vi "GSP_Manager_GT.vi"() -> ()   [LabVIEW 2015]
uses:
  SystemUtil/Command.ctl
  SystemUtil/ScriptArray.ctl
  SystemUtil/Script.ctl
  SystemUtil/MotorStates.ctl
  SystemUtil/ThreadStates.ctl
  Log/LogItem.ctl
  GSP_GT_Global.vi
  GUI/GSP_GUI_global.vi
panel:
  out "Gratings":T1(array[cluster])
  out "lines/mm":i32
  in  "Grating #":i32(ring) items=["<NO GRATING>", "SYZY_400", "RALC_1200", "SYZY_2100"]
  out "Last Error":errorcluster
  in  "CommandQ":string
  # "Grating"
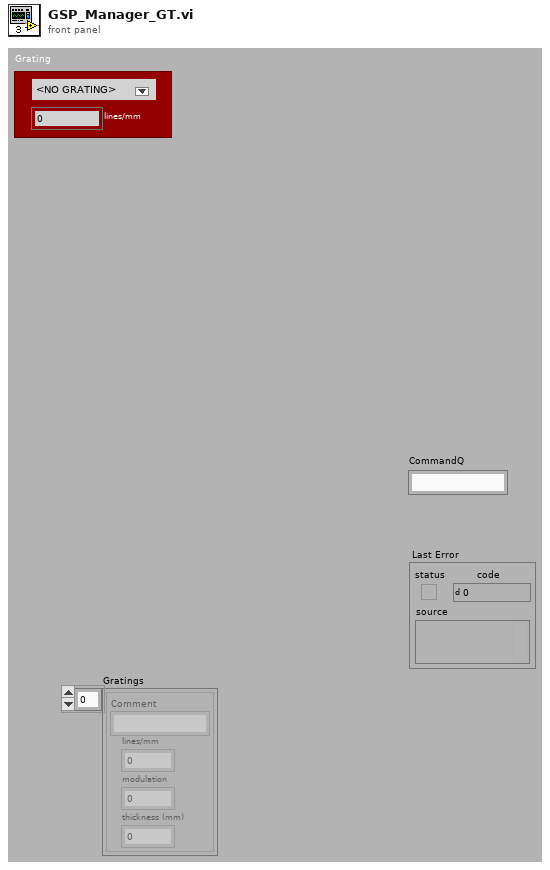
[diagram p1: front panel]
types:
  T1 = cluster{"Comment":string, "lines/mm":i32, "modulation":dbl, "thickness (mm)":dbl}[]
  T2 = typedef "Command.ctl" = cluster{"Command":string, "Parameter":string}
  T3 = typedef "ScriptArray.ctl" = T4[]
  T4 = typedef "Script.ctl" = cluster{"Current Step":i32, "Commands":cluster{"Command":string, "Parameters":string}[]}
  T5 = cluster{"Move Mem Address":i32, "Home Mem Address":i32}
  T6 = typedef "MotorStates.ctl" = enum16{"Ready", "Moving", "Uninitialized", "Error"}
  T7 = typedef "ThreadStates.ctl" = enum16{"Waiting", "Scripting", "Uninitialized", "Error"}
  T8 = cluster{"Comment":string, "lines/mm":i32, "modulation":dbl, "thickness (mm)":dbl}
  T9 = enum16{"Launch", "Log", "Open", "Close", "Shutdown"}
  T10 = typedef "LogItem.ctl" = cluster{"error in (no error)":errorcluster, "Source":string, "Comment ":string}
  T11 = enum16{"POL (0)", "CPL (1)", "HLT (2)", "STP (3)", "RST (4)", "RVN (5)", "RPB (6)", "CLP (8)", "SDL (9)", "RUN (10)", "WRI (11)", "RRG (12)", "SPR (13)", "LPR (14)", "VMI (15)", "SSP (17)", "SSE (18)", "RIS (20)", "RIO (21)", "IMW (25)", "END (128)", "MAV (134)", "MRV (135)", "JRE (137)", "WCL (138)", "WCW (139)", "DLY (140)", "WDL (141)", "GCL (142)", "GOP (143)", "ZTG (144)", "ZTP (145)", "TTP (146)", "CME (147)", "CTC (148)", "TQL (149)", "AHC (150)", "ERL (151)", "OLP (152)", "WRP (154)", "IDT (155)", "LRP (156)", "VMP (159)", "RAV (160)", "RRV (161)", "JMP (162)", "JOI (162)", "CIS (163)", "CKS (164)", "CLC (165)", "KMC (167)", "MCT (168)", "FLC (169)", "EEM (170)", "DDB (171)", "DEM (171)", "PAC (172)", "ADL (173)", "BRT (174)", "MAT (176)", "MRT (177)", "RAT (178)", "RRT (179)", "SSD (180)", "KMR (181)", "KED (182)", "KDD (183)", "DIR (184)", "PRO (185)", "SIF (186)", "EDL (187)", "CIO (188)", "MDS (189)", "MDC (190)", "MDT (191)", "SEE (192)", "ARI (193)", "WBS (194)", "SCF (195)", "RSM (196)", "RLM (197)", "RSN (198)", "RLN (199)", "PCL (201)", "PCI (201)", "PRT (202)", "PRI (202)", "WBE (204)", "SOB (205)", "COB (206)", "ACR (207)", "PLR (208)", "CAI (211)", "LVT (212)", "OVT (213)", "MTT (214)", "CLC (215)", "PIM (216)", "VIM (217)", "TIM (218)", "AHM (219)", "SSL (221)", "TRU (222)", "RSD (223)", "EMT (225)", "DMT (226)", "EMD (227)", "DMD (228)", "HSM (229)", "AHD (230)", "PCM (231)", "PCG (232)", "XRV (233)", "XAV (234)", "XRT (235)", "XAT (236)", "GOC (237)", "JNA (238)", "JOR (239)", "PMC (240)", "PMV (241)", "PMX (242)", "DLC (243)", "SLC (244)", "PCP (245)", "ATR (248)", "PMO (249)", "JAN (250)", "EDH (251)", "DIF (252)", "IMS (253)", "IMQ (254)"}
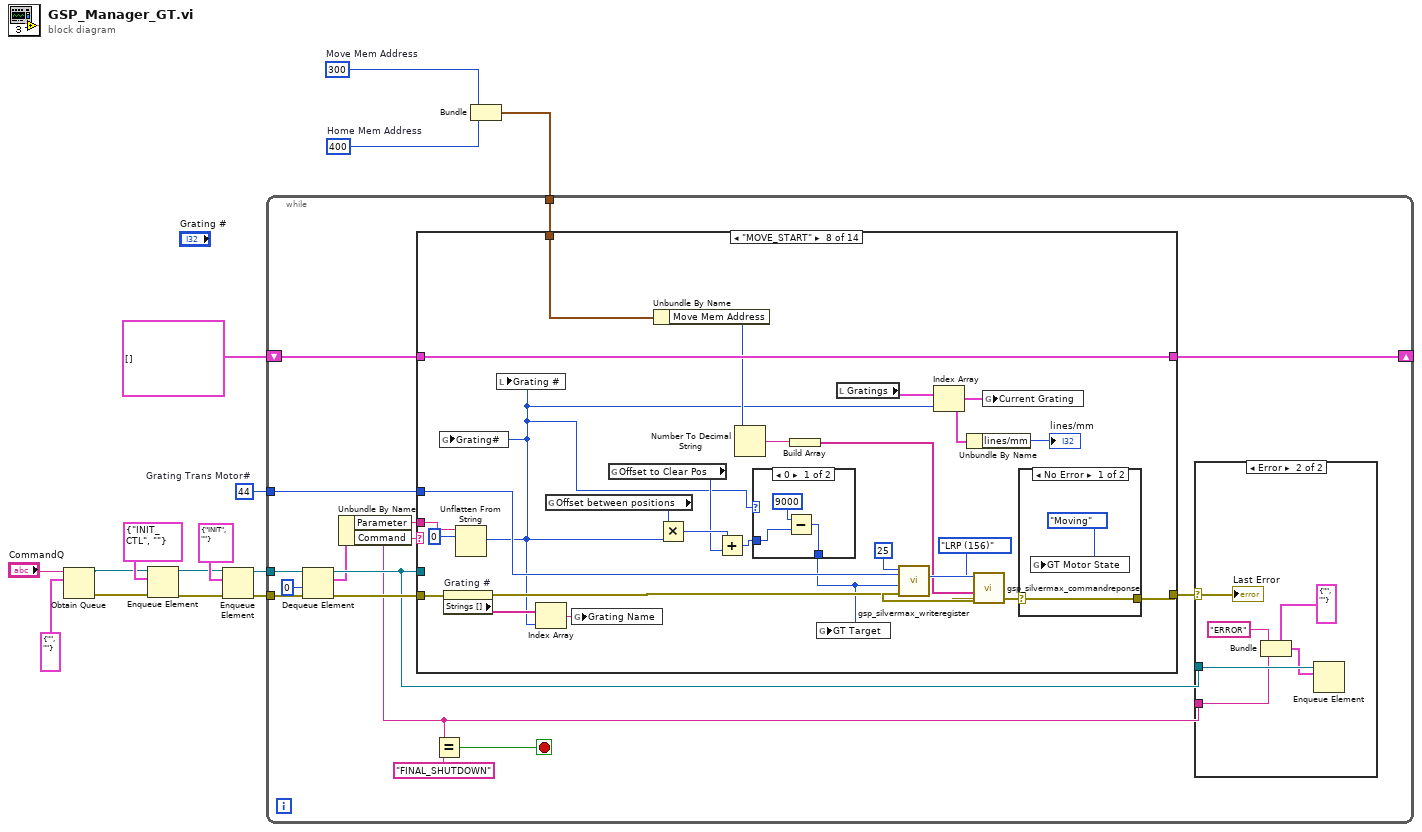
[diagram p0: block diagram]
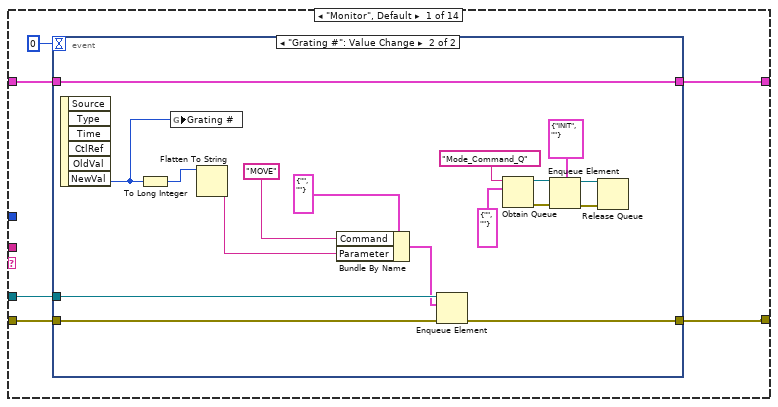
[diagram p3: hidden frame]
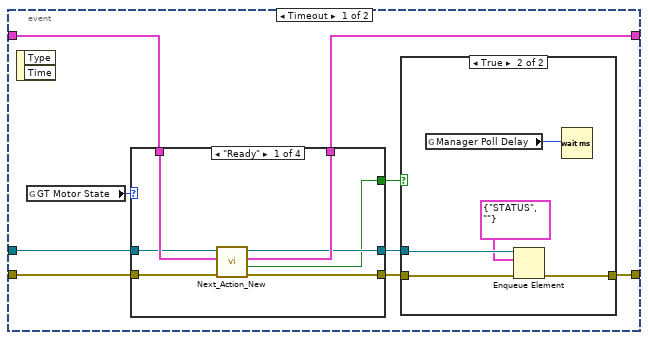
[diagram p4: hidden frame]
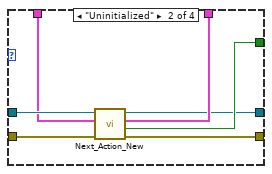
[diagram p6: hidden frame]
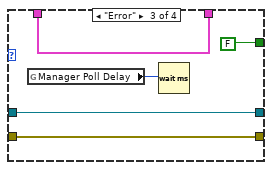
[diagram p7: hidden frame]
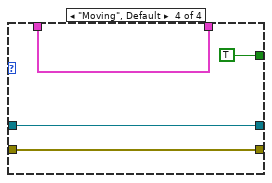
[diagram p8: hidden frame]
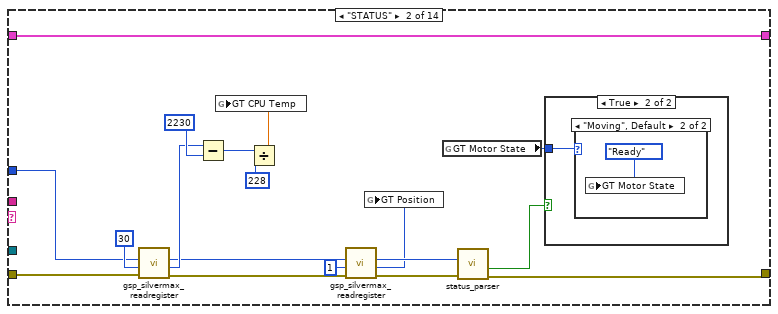
[diagram p9: hidden frame]
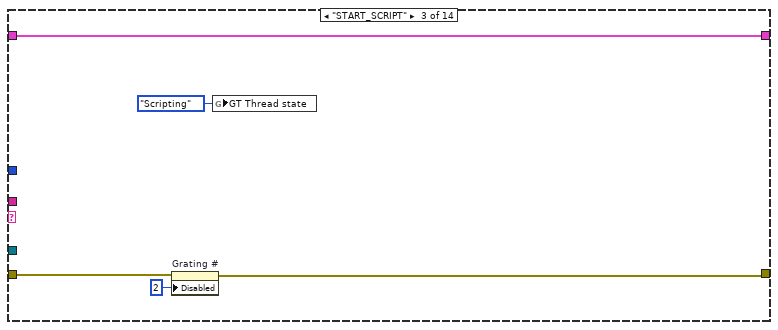
[diagram p12: hidden frame]
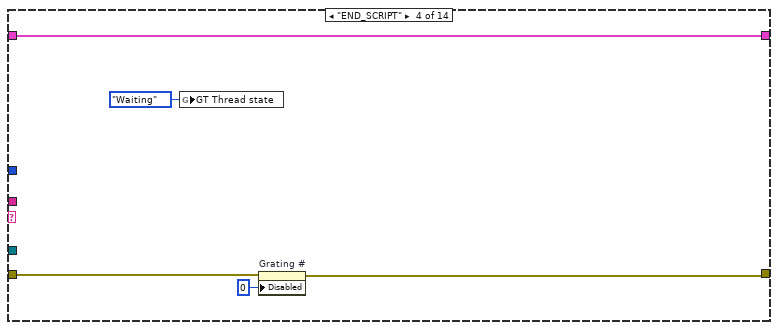
[diagram p13: hidden frame]
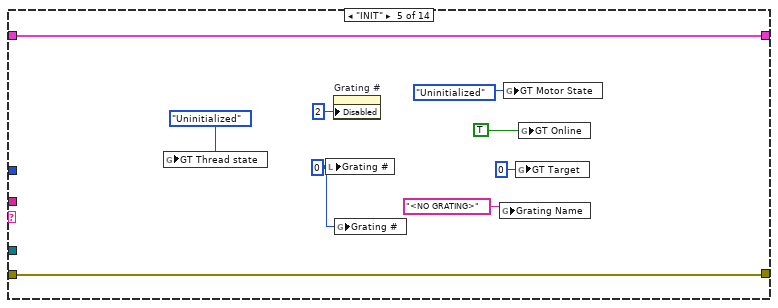
[diagram p14: hidden frame]
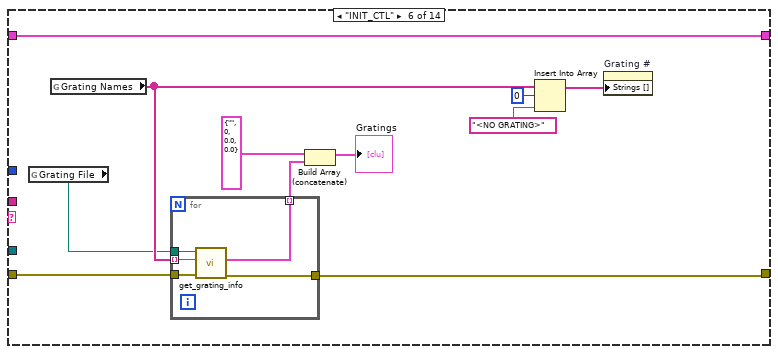
[diagram p15: hidden frame]
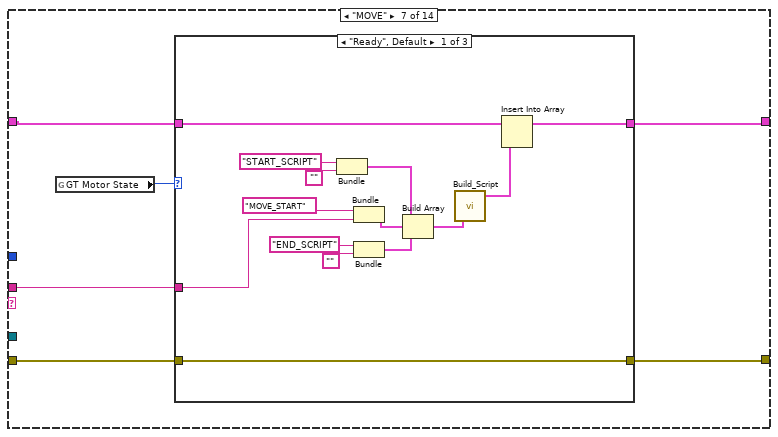
[diagram p16: hidden frame]
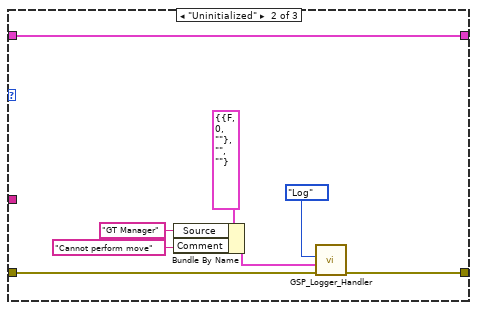
[diagram p17: hidden frame]
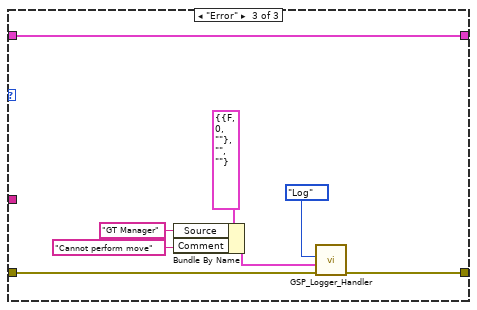
[diagram p18: hidden frame]
diagram:
  w7 = 400  # Home Mem Address
  w8 = 300  # Move Mem Address
  w9 = u8 44  # Grating Trans Motor#
  n1 = Obtain Queue(name (unnamed)="CommandQ", element data type=T2 {"Command"="", "Parameter"=""} ("Command")) -> (queue out=w2:refnum<queue>, error out=w1:errorcluster)  [unwired: 3 in, 1 out]
  n2 = Enqueue Element(queue=w2, element=T2 {"Command"="INIT_CTL", "Parameter"=""}, error in (no error)=w1) -> (queue out=w4:refnum<queue>, error out=w3:errorcluster)  [unwired: 1 in, 1 out]
  n3 = Enqueue Element(queue=w4, element=T2 {"Command"="INIT", "Parameter"=""}, error in (no error)=w3) -> (queue out=w15:refnum<queue>, error out=w14:errorcluster)  [unwired: 1 in, 1 out]
  n4 = Bundle("Move Mem Address"=w8, "Home Mem Address"=w7) -> (w6:T5)  [unwired: 1 in]
  n5 = while {
    tunnel: w15 -> [w30]
    tunnel: w14 -> [w29]
    tunnel: w9 -> [w24]
    shift-right: [w18] -> _
    shift-left: T3 [] ("Operations") -> [w23]
    tunnel: w6 -> [w16]
    stop <- w19 stop-if-true
    n6 = Dequeue Element(queue=w30, timeout in ms (-1)=0, error in (no error)=w29) -> (queue out=w26:refnum<queue>, element=w21:T2, error out=w28:errorcluster)  [unwired: 1 out]
    n7 = Unbundle By Name(w21) -> ("Parameter"=w17:string, "Command"=w20:string)
    n8 = case shown="\"MOVE_START\"" w20 {
      tunnel: w28 -> [w41 w106 w120 w126 w132 w140 w155 w195 w229 w248 w283 w302 w304 _]
      tunnel: w26 -> [w42 _ _ _ _ _ _ _ _ w251 w282 _ _ w326]
      tunnel: [w38 w115 w119 w125 w132 w143 w154 w209 w237 w250 w279 w302 w312 _] -> w27
      tunnel: w24 -> [_ w105 _ _ _ _ _ w212 w240 _ _ _ w314 _]
      tunnel: w23 -> [w40 w113 w122 w127 w135 w147 w158 w206 w234 w252 w281 w301 w309 w320]
      tunnel: [w39 w113 w122 w127 w135 w147 w157 w206 w234 w249 w281 w300 w309 w319] -> w18
      tunnel: w17 -> [_ _ _ _ _ _ w156 w205 _ _ _ _ _ _]
      tunnel: w16 -> [_ _ _ _ _ _ _ w200 w233 _ _ _ w307 _]
      frame "Monitor", Default {
        n9 = event shown="[1] \"Grating #\": Value Change" {
          selector: _ -> [_ _]
          dyn-events: _ -> [_ _]
          timeout: 0 -> [_ _]
          tunnel: w42 -> [w51 w90]
          tunnel: w41 -> [w50 w91]
          tunnel: w40 -> [w49 w97]
          tunnel: [w48 w97] -> w39
          tunnel: [w44 w92] -> w38
          event Timeout {
            n10 = event-data() -> ()  [unwired: 1 in, 2 out]
            n11 = global read "GSP_GT_Global.vi" "GT Motor State"() -> (w43:T6)
            n12 = case shown="\"Ready\"" w43 {
              tunnel: w51 -> [w60 w69 w73 w78]
              tunnel: w50 -> [w64 w71 w75 w79]
              tunnel: [w62 w70 w75 w79] -> w47
              tunnel: w49 -> [w61 w68 w74 w80]
              tunnel: [w63 w67 w74 w80] -> w48
              tunnel: [w59 w65 w73 w78] -> w46
              tunnel: [w58 w66 FALSE TRUE] -> w45
              frame "Ready" {
                n13 = call "Next_Action_New.vi"("error in (no error)"=w64, "Operations"=w61, "queue in"=w60) -> ("error out"=w62:errorcluster, "No command?"=w58:bool, "Operations Out"=w63:T3, "queue out"=w59:refnum<queue>)  [unwired: 1 in]
              }
              frame "Uninitialized" {
                n14 = call "Next_Action_New.vi"("error in (no error)"=w71, "Operations"=w68, "queue in"=w69) -> ("error out"=w70:errorcluster, "No command?"=w66:bool, "Operations Out"=w67:T3, "queue out"=w65:refnum<queue>)  [unwired: 1 in]
              }
              frame "Error" {
                n15 = global read "GSP_GUI_global.vi" "Manager Poll Delay"() -> (w76:u32)
                n16 = Wait (ms)(milliseconds to wait=w76) -> ()  [unwired: 1 out]
              }
              frame "Moving", Default {
              }
            }
            n17 = case shown="True" w45 {
              tunnel: w47 -> [w52 w57]
              tunnel: w46 -> [_ w56]
              tunnel: [w52 w55] -> w44
              frame False {
              }
              frame True {
                n18 = global read "GSP_GUI_global.vi" "Manager Poll Delay"() -> (w54:u32)
                n19 = Enqueue Element(queue=w56, element=T2 {"Command"="STATUS", "Parameter"=""}, error in (no error)=w57) -> (error out=w55:errorcluster)  [unwired: 1 in, 2 out]
                n20 = Wait (ms)(milliseconds to wait=w54) -> ()  [unwired: 1 out]
              }
            }
          }
          event "Grating #": Value Change {
            n21 = event-data() -> ("NewVal"=w88:i32)  [unwired: 1 in, 5 out]
            n22 = To Long Integer(number=w88) -> (32bit integer=w93:i32)
            n23 = global write "GSP_GT_Global.vi" "Grating #"(w88) -> ()
            n24 = Flatten To String(anything=w93) -> (data string=w94:string)  [unwired: 3 in, 2 out]
            n25 = Bundle By Name(cluster=T2 {"Command"="", "Parameter"=""} ("Command"), "Command"="MOVE" ("element"), "Parameter"=w94) -> (w89:T2)
            n26 = Enqueue Element(queue=w90, element=w89, error in (no error)=w91) -> (error out=w92:errorcluster)  [unwired: 1 in, 2 out]
            n27 = Obtain Queue(name (unnamed)="Mode_Command_Q", element data type=T2 {"Command"="", "Parameter"=""} ("element")) -> (queue out=w87:refnum<queue>, error out=w86:errorcluster)  [unwired: 3 in, 1 out]
            n28 = Enqueue Element(queue=w87, element=T2 {"Command"="INIT", "Parameter"=""}, error in (no error)=w86) -> (queue out=w82:refnum<queue>, error out=w81:errorcluster)  [unwired: 1 in, 1 out]
            n29 = Release Queue(queue=w82, error in (no error)=w81) -> ()  [unwired: 1 in, 3 out]
          }
        }
      }
      frame "STATUS" {
        n30 = call "gsp_silvermax_readregister.vi"("error in (no error)"=w106, "Register# (0)"=u8 30, "Motor #"=w105) -> ("error out"=w103:errorcluster, "Register Value"=w111:i32, "Motor # dup"=w102:u8)  [unwired: 2 in, 2 out]
        n31 = Subtract(x=w111, y=2230) -> (x-y=w110:i32)
        n32 = Divide(x=w110, y=228) -> (x/y=w107:dbl)
        n33 = global write "GSP_GT_Global.vi" "GT CPU Temp"(w107) -> ()
        n34 = call "gsp_silvermax_readregister.vi"("error in (no error)"=w103, "Register# (0)"=u8 1, "Motor #"=w102) -> ("error out"=w104:errorcluster, "Register Value"=w99:i32, "Motor # dup"=w100:u8)  [unwired: 2 in, 2 out]
        n35 = global write "GSP_GT_Global.vi" "GT Position"(w99) -> ()
        n36 = global read "GSP_GT_Global.vi" "GT Motor State"() -> (w98:T6)
        n37 = call "status_parser.vi"("error in (no error)"=w104, "Motor #"=w100) -> ("error out"=w115:errorcluster, "Program Complete?"=w114:bool)  [unwired: 3 in, 1 out]
        n38 = case shown="True" w114 {
          tunnel: w98 -> [_ w116]
          frame False {
          }
          frame True {
            n39 = case shown="\"Moving\", Default" w116 {
              frame "Uninitialized" {
              }
              frame "Moving", Default {
                n40 = global write "GSP_GT_Global.vi" "GT Motor State"(MotorStates."Ready" ("Mode")) -> ()
              }
            }
          }
        }
      }
      frame "START_SCRIPT" {
        n41 = property on="Grating #" class="Ring (strict)"(error in=w120, "Disabled"=u8 2) -> (error out=w119:errorcluster)  [unwired: 1 in, 1 out]
        n42 = global write "GSP_GT_Global.vi" "GT Thread state"(ThreadStates."Scripting" ("GT Thread state")) -> ()
      }
      frame "END_SCRIPT" {
        n43 = global write "GSP_GT_Global.vi" "GT Thread state"(ThreadStates."Waiting" ("GT Thread state")) -> ()
        n44 = property on="Grating #" class="Ring (strict)"(error in=w126, "Disabled"=u8 0) -> (error out=w125:errorcluster)  [unwired: 1 in, 1 out]
      }
      frame "INIT" {
        w128 = 0 ("Value")
        n45 = global write "GSP_GT_Global.vi" "GT Thread state"(ThreadStates."Uninitialized" ("Thread state")) -> ()
        n46 = local write "Grating #"(w128) -> ()
        n47 = property on="Grating #" class="Ring (strict)"("Disabled"=u8 2) -> ()  [unwired: 2 in, 2 out]
        n48 = global write "GSP_GT_Global.vi" "Grating #"(w128) -> ()
        n49 = global write "GSP_GT_Global.vi" "Grating Name"("<NO GRATING>" ("new element/subarray")) -> ()
        n50 = global write "GSP_GT_Global.vi" "GT Motor State"(MotorStates."Uninitialized" ("Mode")) -> ()
        n51 = global write "GSP_GT_Global.vi" "GT Target"(0 ("GT Target")) -> ()
        n52 = global write "GSP_GT_Global.vi" "GT Online"(TRUE ("CS Online")) -> ()
      }
      frame "INIT_CTL" {
        n53 = global read "GSP_GUI_global.vi" "Grating File"() -> (w141:path)
        n54 = global read "GSP_GUI_global.vi" "Grating Names"() -> (w142:string[])
        n55 = for {
          tunnel: [w152] -> w139 mode=indexing
          tunnel: [w151] -> w143
          tunnel: w142 -> [w150] mode=indexing
          tunnel: w141 -> [w149]
          tunnel: w140 -> [w148]
          n56 = call "get_grating_info.vi"("error in (no error)"=w148, "grating name"=w150, "configuration file path"=w149) -> ("error out"=w151:errorcluster, "Grating Info"=w152:T8)  [unwired: 3 in]
        }
        n57 = Build Array (concatenate)(T8 {"Comment"="", "lines/mm"=0, "modulation"=0.0, "thickness (mm)"=0.0} ("Grating Info"), w139) -> (→"Gratings":T1)
        n58 = Insert Into Array(array=w142, index=0, new element="<NO GRATING>" ("new element/subarray")) -> (w144:string[])
        n59 = property on="Grating #" class="Ring (strict)"("Strings []"=w144) -> ()  [unwired: 2 in, 2 out]
      }
      frame "MOVE" {
        n60 = global read "GSP_GT_Global.vi" "GT Motor State"() -> (w153:T6)
        n61 = case shown="\"Ready\", Default" w153 {
          tunnel: w158 -> [w172 w180 w188]
          tunnel: [w171 w180 w188] -> w157
          tunnel: w156 -> [w168 _ _]
          tunnel: w155 -> [w170 w179 w187]
          tunnel: [w170 w178 w186] -> w154
          frame "Ready", Default {
            n62 = Bundle("START_SCRIPT", "") -> (w159:cluster{string, string})  [unwired: 1 in]
            n63 = Bundle("MOVE_START", "Parameter"=w168) -> (w165:cluster{string, "Parameter":string})  [unwired: 1 in]
            n64 = Bundle("END_SCRIPT", "") -> (w164:cluster{string, string})  [unwired: 1 in]
            n65 = Build Array(w159, w165, w164) -> (w163:cluster{string, "Parameter":string}[])
            n66 = call "Build_Script.vi"("Commands"=w163) -> ("script out"=w162:T4)  [unwired: 4 in]
            n67 = Insert Into Array(array=w172, new element=w162) -> (w171:T3)  [unwired: 1 in]
          }
          frame "Uninitialized" {
            n68 = Bundle By Name(cluster=T10 {"error in (no error)"={"status"=FALSE, "code"=0, "source"=""}, "Source"="", "Comment "=""} ("Log"), "Source"="GT Manager", "Comment"="Cannot perform move") -> (w176:T10)
            n69 = call "GSP_Logger_Handler.vi"("error in (no error)"=w179, "Log"=w176, "Actions"=T9."Log") -> ("error out"=w178:errorcluster)  [unwired: 4 in]
          }
          frame "Error" {
            n70 = Bundle By Name(cluster=T10 {"error in (no error)"={"status"=FALSE, "code"=0, "source"=""}, "Source"="", "Comment "=""} ("Log"), "Source"="GT Manager", "Comment"="Cannot perform move") -> (w184:T10)
            n71 = call "GSP_Logger_Handler.vi"("error in (no error)"=w187, "Log"=w184, "Actions"=T9."Log") -> ("error out"=w186:errorcluster)  [unwired: 4 in]
          }
        }
      }
      frame "MOVE_START" {
        n72 = property on="Grating #" class="Ring (strict)"(error in=w195) -> (error out=w193:errorcluster, "Strings []"=w194:string[])  [unwired: 1 in, 1 out]
        n73 = Unflatten From String(type=0, binary string=w205) -> (value=w189:i32)  [unwired: 3 in, 2 out]
        n74 = global write "GSP_GT_Global.vi" "Grating#"(w189) -> ()
        n75 = local write "Grating #"(w189) -> ()
        n76 = Index Array(array=w194, index=w189) -> (element=w192:string)
        n77 = global read "GSP_GT_Global.vi" "Offset between positions"() -> (w203:i32)
        n78 = global write "GSP_GT_Global.vi" "Grating Name"(w192) -> ()
        n79 = global read "GSP_GT_Global.vi" "Offset to Clear Pos"() -> (w201:i32)
        n80 = Unbundle By Name(w200) -> ("Move Mem Address"=w199:i32)
        n81 = Multiply(x=w203, y=w189) -> (x*y=w202:i32)
        n82 = Add(x=w202, y=w201) -> (x+y=w191:i32)
        n83 = Number To Decimal String(number=w199) -> (decimal integer string=w208:string)  [unwired: 1 in]
        n84 = case shown="0" w189 {
          tunnel: w191 -> [w218 w219]
          tunnel: [w217 w219] -> w190
          frame 0 {
            n85 = Subtract(x=9000, y=w218) -> (x-y=w217:i32)
          }
          frame Default {
          }
        }
        n86 = Build Array(w208) -> (w207:string[])
        n87 = global write "GSP_GT_Global.vi" "GT Target"(w190) -> ()
        n88 = local read "Gratings"() -> (w198:T1)
        n89 = call "gsp_silvermax_writeregister.vi"("error in (no error)"=w193, "Register Value"=w190, "Motor #"=w212, "Register# (0)"=u8 25) -> ("error out"=w214:errorcluster, "Motor # dup"=w213:u8)  [unwired: 2 in]
        n90 = Index Array(array=w198, index=w189) -> (element=w197:T8)
        n91 = Unbundle By Name(w197) -> ("lines/mm"=→"lines/mm":i32)
        n92 = call "gsp_silvermax_commandreponse.vi"("error in (no error)"=w214, "Parameters (none)"=w207, "Motor #"=w213, "Command"=T11."LRP (156)") -> ("error out"=w210:errorcluster)  [unwired: 3 out]
        n93 = global write "GSP_GT_Global.vi" "Current Grating"(w197) -> ()
        n94 = case shown="No Error" w210 {
          selector: w210 -> [w221 w222]
          tunnel: [w221 w222] -> w209
          frame No Error {
            n95 = global write "GSP_GT_Global.vi" "GT Motor State"(MotorStates."Moving" ("Mode")) -> ()
          }
          frame Error {
          }
        }
      }
      frame "MOVE_DETENT" {
        w224 = -400 ("GT Target")
        w225 = 0
        n96 = global write "GSP_GT_Global.vi" "Grating#"(w225) -> ()
        n97 = property on="Grating #" class="Ring (strict)"(error in=w229) -> (error out=w227:errorcluster, "Strings []"=w228:string[])  [unwired: 1 in, 1 out]
        n98 = local write "Grating #"(w225) -> ()
        n99 = Index Array(array=w228, index=w225) -> (element=w226:string)
        n100 = global write "GSP_GT_Global.vi" "Grating Name"(w226) -> ()
        n101 = Unbundle By Name(w233) -> ("Move Mem Address"=w232:i32)
        n102 = global write "GSP_GT_Global.vi" "GT Target"(w224) -> ()
        n103 = Number To Decimal String(number=w232) -> (decimal integer string=w236:string)  [unwired: 1 in]
        n104 = call "gsp_silvermax_writeregister.vi"("error in (no error)"=w227, "Register Value"=w224, "Motor #"=w240, "Register# (0)"=u8 25) -> ("error out"=w242:errorcluster, "Motor # dup"=w241:u8)  [unwired: 2 in]
        n105 = Build Array(w236) -> (w235:string[])
        n106 = call "gsp_silvermax_commandreponse.vi"("error in (no error)"=w242, "Parameters (none)"=w235, "Motor #"=w241, "Command"=T11."LRP (156)") -> ("error out"=w238:errorcluster)  [unwired: 3 out]
        n107 = local read "Gratings"() -> (w231:T1)
        n108 = case shown="No Error" w238 {
          selector: w238 -> [w245 w246]
          tunnel: [w245 w246] -> w237
          frame No Error {
            n109 = global write "GSP_GT_Global.vi" "GT Motor State"(MotorStates."Moving" ("Mode")) -> ()
          }
          frame Error {
          }
        }
        n110 = Index Array(array=w231, index=w225) -> (element=w230:T8)
        n111 = Unbundle By Name(w230) -> ("lines/mm"=w223:i32)
        n112 = global write "GSP_GT_Global.vi" "Current Grating"(w230) -> ()
        n113 = local write "lines/mm"(w223) -> ()
      }
      frame "SHUTDOWN" {
        n114 = global read "GSP_GT_Global.vi" "GT Motor State"() -> (w247:T6)
        n115 = case shown="\"Ready\", Default" w247 {
          tunnel: [w268 w272 w276] -> w249
          tunnel: w252 -> [w267 w272 w276]
          tunnel: w251 -> [_ w271 w275]
          tunnel: [w263 w269 w273] -> w250
          tunnel: w248 -> [w263 _ _]
          frame "Ready", Default {
            w259 = ""
            n116 = Bundle("START_SCRIPT", "") -> (w257:cluster{string, string})  [unwired: 1 in]
            n117 = Bundle("MOVE_DETENT", w259) -> (w256:cluster{string, string})  [unwired: 1 in]
            n118 = Bundle("FINAL_SHUTDOWN", "") -> (w254:cluster{string, string})  [unwired: 1 in]
            n119 = Bundle("END_SCRIPT", w259) -> (w255:cluster{string, string})  [unwired: 1 in]
            n120 = Build Array(w257, w256, w255, w254) -> (w253:cluster{string, string}[])
            n121 = call "Build_Script.vi"("Commands"=w253) -> ("script out"=w266:T4)  [unwired: 4 in]
            n122 = Insert Into Array(array=w267, new element=w266) -> (w268:T3)  [unwired: 1 in]
          }
          frame "Uninitialized" {
            n123 = Enqueue Element(queue=w271, element=T2 {"Command"="FINAL_SHUTDOWN", "Parameter"=""}) -> (error out=w269:errorcluster)  [unwired: 2 in, 2 out]
          }
          frame "Error" {
            n124 = Enqueue Element(queue=w275, element=T2 {"Command"="FINAL_SHUTDOWN", "Parameter"=""}) -> (error out=w273:errorcluster)  [unwired: 2 in, 2 out]
          }
        }
      }
      frame "FINAL_SHUTDOWN" {
        n125 = Release Queue(queue=w282, error in (no error)=w283) -> (error out=w277:errorcluster)  [unwired: 1 in, 2 out]
        n126 = global write "GSP_GT_Global.vi" "GT Thread state"(ThreadStates."Uninitialized" ("Thread state")) -> ()
        n127 = property on="Grating #" class="Ring (strict)"(error in=w277, "Disabled"=u8 2) -> (error out=w279:errorcluster)  [unwired: 1 in, 1 out]
        n128 = stacked-sequence {
          tunnel: w279 -> [_]
          frame #0 {
            n129 = global write "GSP_GT_Global.vi" "GT Online"(FALSE ("CS Online")) -> ()
          }
        }
      }
      frame "HOME" {
        n130 = Flatten To String(anything=0) -> (data string=w295:string)  [unwired: 3 in, 2 out]
        n131 = Bundle("START_SCRIPT", "") -> (w285:cluster{string, string})  [unwired: 1 in]
        n132 = Bundle("END_SCRIPT", "") -> (w290:cluster{string, string})  [unwired: 1 in]
        n133 = Bundle("HOME_START", "") -> (w292:cluster{string, string})  [unwired: 1 in]
        n134 = Bundle("MOVE_START", "data string"=w295) -> (w291:cluster{string, "data string":string})  [unwired: 1 in]
        n135 = Build Array(w285, w292, w291, w290) -> (w289:cluster{string, "data string":string}[])
        n136 = call "Build_Script.vi"("Commands"=w289) -> ("script out"=w288:T4)  [unwired: 4 in]
        n137 = Insert Into Array(array=w301, new element=w288) -> (w300:T3)  [unwired: 1 in]
      }
      frame "HOME_START" {
        n138 = Unbundle By Name(w307) -> ("Home Mem Address"=w306:i32)
        n139 = global write "GSP_GT_Global.vi" "Grating Name"("<NO GRATING>" ("new element/subarray")) -> ()
        n140 = local write "Grating #"(0 ("Value")) -> ()
        n141 = Number To Decimal String(number=w306) -> (decimal integer string=w311:string)  [unwired: 1 in]
        n142 = Build Array(w311) -> (w310:string[])
        n143 = call "gsp_silvermax_commandreponse.vi"("error in (no error)"=w304, "Parameters (none)"=w310, "Motor #"=w314, "Command"=T11."LRP (156)") -> ("error out"=w315:errorcluster)  [unwired: 3 out]
        n144 = case shown="No Error" w315 {
          selector: w315 -> [w317 w318]
          tunnel: [w317 w318] -> w312
          frame No Error {
            n145 = global write "GSP_GT_Global.vi" "GT Motor State"(MotorStates."Moving" ("Mode")) -> ()
          }
          frame Error {
          }
        }
        n146 = global write "GSP_GT_Global.vi" "GT Target"(0 ("GT Target")) -> ()
      }
      frame "ERROR" {
        n147 = local read "Last Error"() -> (w322:errorcluster)
        n148 = Unbundle By Name(w322) -> ("code"=w328:i32)
        n149 = Bundle By Name(cluster=T10 {"error in (no error)"={"status"=FALSE, "code"=0, "source"=""}, "Source"="", "Comment "=""} ("Log"), "error in (no error)"=w322, "Source"="GT Manager") -> (w323:T10)
        n150 = call "GSP_Logger_Handler.vi"("Log"=w323, "Actions"=T9."Log") -> ()  [unwired: 5 in, 1 out]
        n151 = case shown="5003, 5006" w328 {
          tunnel: w322 -> [_ _ _]
          tunnel: [errorcluster {"status"=FALSE, "code"=0, "source"=""} ("Last Error") errorcluster {"status"=FALSE, "code"=0, "source"=""} ("Last Error") errorcluster {"status"=FALSE, "code"=0, "source"=""} ("Last Error")] -> w327
          tunnel: w320 -> [_ w337 w339]
          tunnel: [T3 [] ("Operations") w337 w339] -> w319
          frame 0, Default {
            n152 = global write "GSP_GT_Global.vi" "GT Motor State"(MotorStates."Error" ("Mode")) -> ()
            n153 = global write "GSP_GT_Global.vi" "GT Thread state"(ThreadStates."Error" ("GT Thread state")) -> ()
            n154 = property on="Grating #" class="Ring (strict)"("Disabled"=u8 2) -> ()  [unwired: 2 in, 2 out]
          }
          frame 5003, 5006 {
          }
          frame 5013 {
          }
        }
        n155 = case shown="Error" w327 {
          tunnel: w326 -> [_ w330]
          frame No Error {
          }
          frame Error {
            n156 = Enqueue Element(queue=w330, element=T2 {"Command"="FINAL_SHUTDOWN", "Parameter"=""}) -> ()  [unwired: 2 in, 3 out]
          }
        }
      }
    }
    n157 = Equal?(x=w20, y="FINAL_SHUTDOWN") -> (x = y?=w19:bool)
    n158 = case shown="Error" w27 {
      selector: w27 -> [_ w35]
      tunnel: w26 -> [_ w36]
      tunnel: w20 -> [_ w33]
      frame No Error {
      }
      frame Error {
        n159 = Bundle(cluster=T2 {"Command"="", "Parameter"=""} ("element"), "Command"="ERROR" ("element"), "Parameter"=w33) -> (w32:T2)
        n160 = Enqueue Element(queue=w36, element=w32) -> ()  [unwired: 2 in, 3 out]
        "Last Error" <- w35
      }
    }
  }
